vi "ACOPLADORES.vi"() -> ()   [LabVIEW 2014]
uses:
  <vilib>/Platform/TimedLoop/XDataNode/timing_clust.ctl
  <vilib>/Platform/TimedLoop/XDataNode/nitl_modes.ctl
  <vilib>/Platform/TimedLoop/XDataNode/wakeup.ctl
  <vilib>/Instr/_visa.llb/VISA Configure Serial Port (Instr).vi
  <vilib>/Platform/TimedLoop/XDataNode/XDataNode.xnode
  <userlib>/Newport ESP301/Newport ESP301.lvlib
  <vilib>/Platform/TimedLoop/XDataNode/XDNodeRunTimeDep.lvlib
panel:
  in  "Aceleração":dbl=300.0
  in  "D (um)":dbl=100.0
  in  "Raio":dbl=80.0
  in  "l int":dbl=50.0
  in  "Velocity":dbl=2.0
  out "PROGRESSÃO":i32=8
  in  "N_Guias":u32=8
  in  "Iniciar":bool
  in  "L":dbl=14.0 format="%.1f"
  in  "In.Curva":dbl=1.0
  in  "d (um)":dbl=7.0
  in  "Stop Button":bool
  out "X (mm)":dbl format="%.2g"
  out "Y (um)":dbl format="%.1f"
  out "XY Graph":cluster{dbl[], dbl[]}(graph)
  in  "Refresh Button":bool
  # "Tam.amostra (mm)"
  # "Núm.Acoplad."
  # "Inicio curva"
  # "Raio"
  # "D.Comp.Int. (um)"
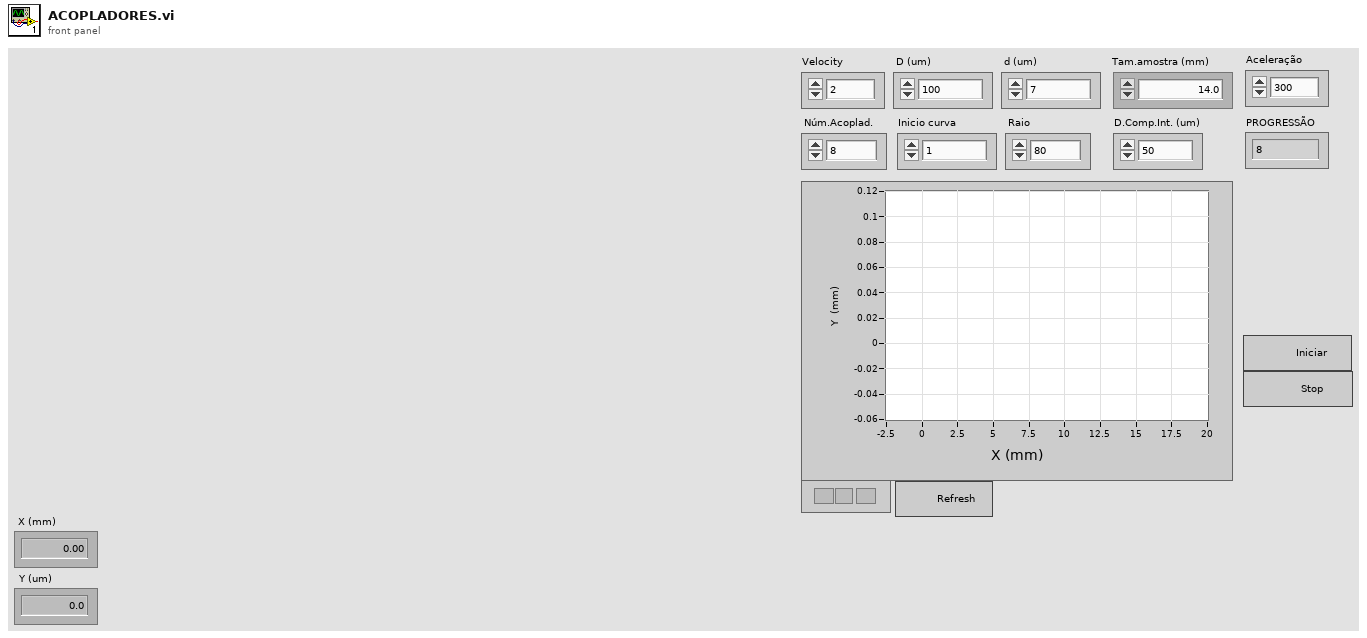
[diagram p1: front panel]
types:
  T1 = typedef "XDNodeRunTimeDep.lvlib/timing_clust.ctl" = cluster{"Expected End [f-1]":u64, "Actual End [f-1]":u64, "Finished Late? [f-1]":bool, "Expected End [i-1]":u64, "Actual End [i-1]":u64, "Finished Late? [i-1]":bool, "Expected Start [i]":u64, "Actual Start [i]":u64, "Expected Start [f]":u64, "Actual Start [f]":u64, "Source Name":string, "Structure Name":string, "Period":i64, "Deadline":i64, "Offset":i64, "Start":i64, "Priority":i32, "Timeout":i32, "Mode":T2, "Wakeup Reason":T3, "Error":errorcluster, "Source Type":string, "Secondary Source Type":string, "Global End Time":u64, "Global Start Time":u64, "Frame Duration":u64, "Iteration Duration":u64, "Assigned CPU":i32, "I/O Scan Engine Mode":u32}
  T2 = typedef "XDNodeRunTimeDep.lvlib/nitl_modes.ctl" = enum32{"No Change", "Process missed periods, maintain original phase", "Discard missed periods, maintain original phase", "Process missed periods, ignore original phase", "Discard missed periods, ignore original phase"}
  T3 = typedef "XDNodeRunTimeDep.lvlib/wakeup.ctl" = enum32{"Normal", "Aborted", "Asynchronous wakeup", "Timing source error", "Timed loop error", "Timeout"}
  T4 = cluster{"Axis1 moving":bool, "Axis2 moving":bool, "Axis3 moving":bool, "Axis4 moving":bool, "Motor Power of at least one axis":bool, "Reserved":bool, "Reserved":bool, "Reserved":bool, "Axis5 moving 2":bool, "Axis6 moving 2":bool, "Reserved":bool, "Reserved":bool, "Motor Power of at least one axis":bool, "Reserved":bool, "Reserved":bool, "Reserved":bool}
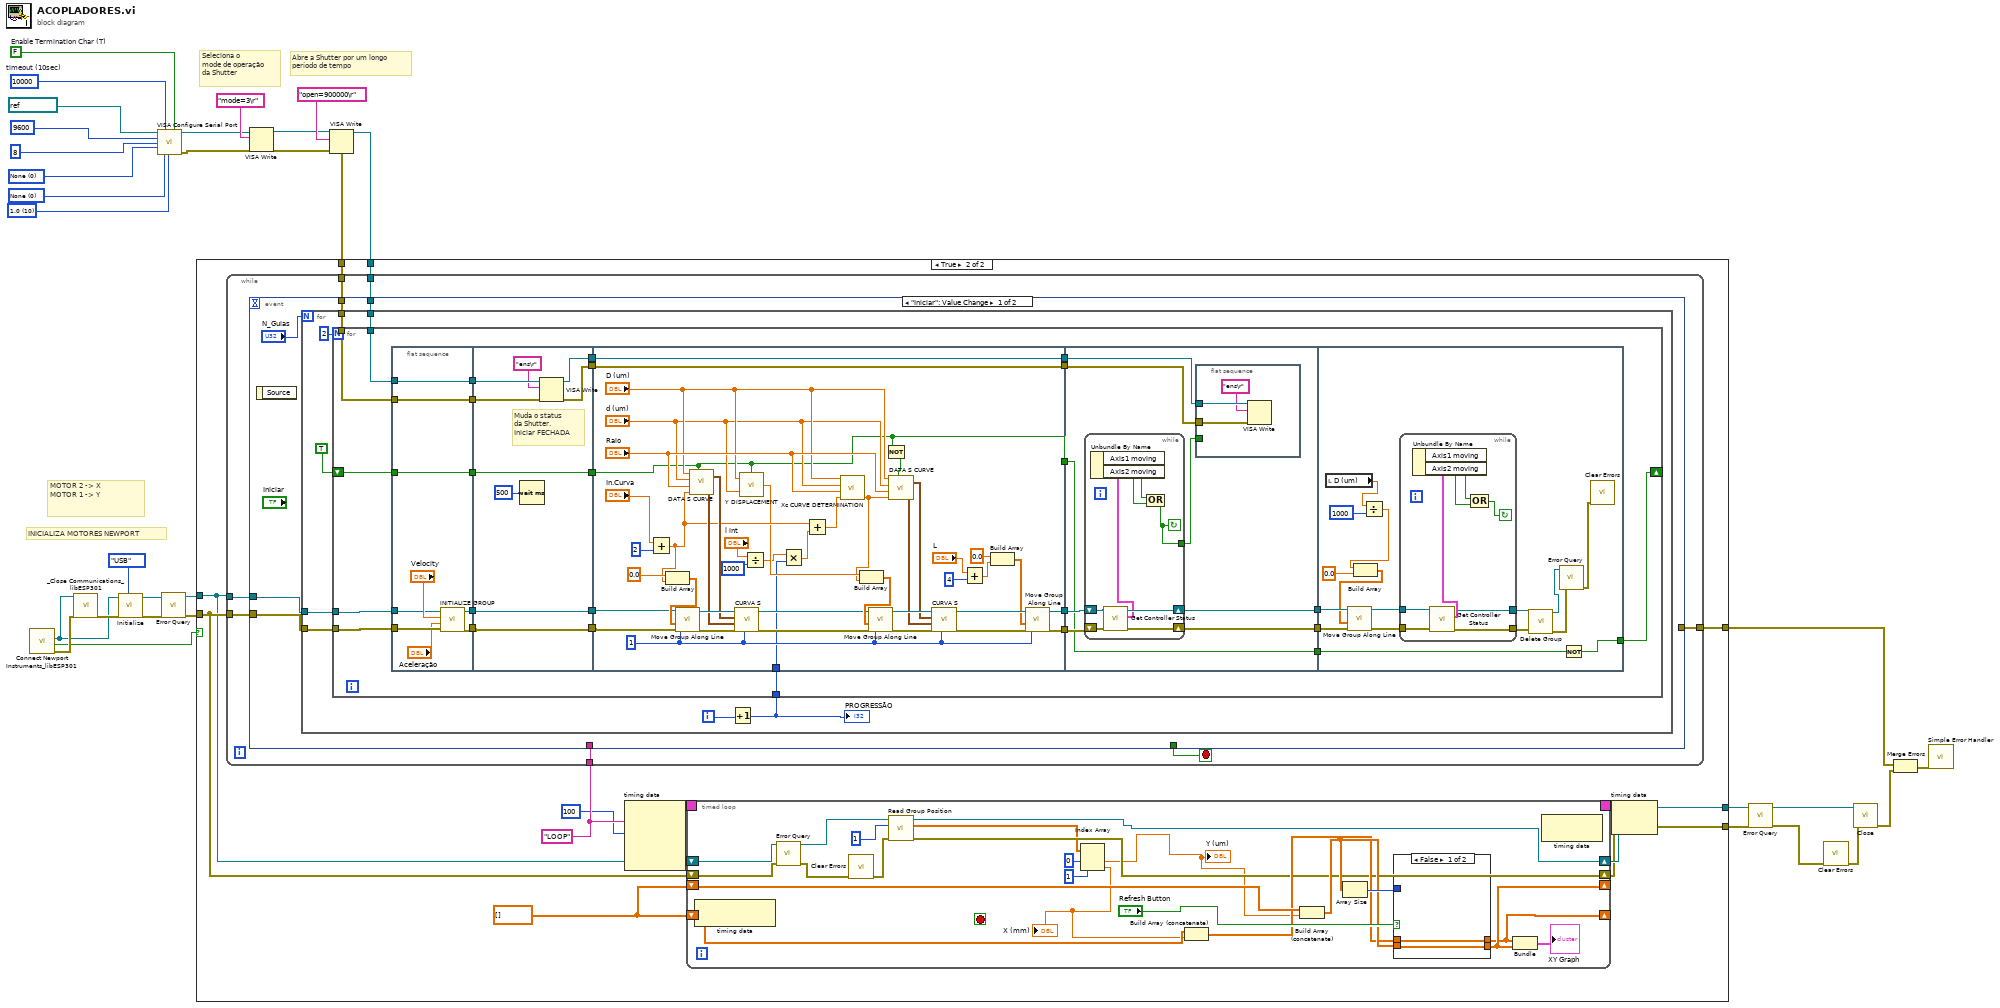
[diagram p0: block diagram]
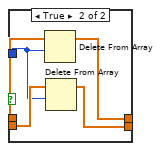
[diagram p3: hidden frame]
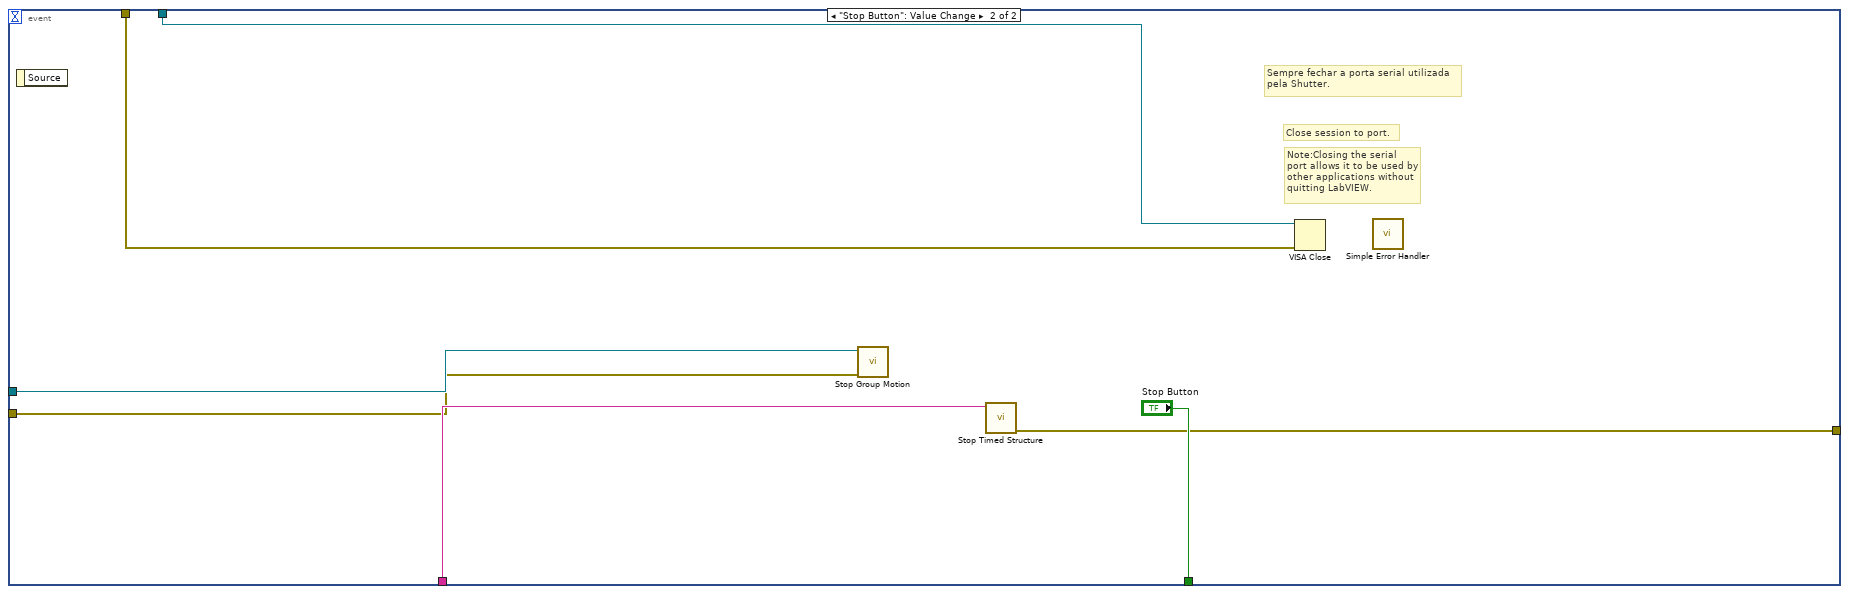
[diagram p4: hidden frame]
diagram:
  w9 = u16 0 items=["None", "Odd", "Even", "Mark", "Space"] ("parity")
  w12 = u16 10 items=["1.0"=10, "1.5"=15, "2.0"=20] ("stop bits")
  w13 = u16 0 items=["None"=0, "XON/XOFF"=1, "RTS/CTS"=2, "DTR/DSR"=4] ("flow control")
  w11 = FALSE  # Enable Termination Char (T)
  w10 = u32 10000  # timeout (10sec)
  # "Abre a Shutter por um longo\nperíodo de tempo"
  # "Seleciona o \nmode de operação\nda Shutter"
  # "MOTOR 2 -> X\nMOTOR 1 -> Y"
  # "INICIALIZA MOTORES NEWPORT"
  n1 = call <userlib>:"Connect Newport Instruments_libESP301.vi"() -> ("error (duplicate)"=w31:errorcluster, "Connected"=w20:bool, "VISA resource name (duplicate)"=w30:refnum<visa-resource-name>)  [unwired: 7 in, 2 out]
  n2 = call <userlib>:"_Close Communications_libESP301.vi"("Instrument Channel"=w30, "error in (no error)"=w31) -> ("error out"=w33:errorcluster)  [unwired: 13 in]
  n3 = call <userlib>:"Initialize.vi"("VISA resource name"=w30, "error in (no error)"=w33, "Serial Link (RS232)"=enum16{"RS232", "USB"}."USB") -> ("VISA resource name out"=w29:refnum<visa-resource-name>, "error out"=w28:errorcluster)  [unwired: 6 in]
  n4 = call-poly "VISA Configure Serial Port"("VISA resource name"=refnum<visa-resource-name> "COM6", "timeout (10sec)"=w10, "Enable Termination\nChar (T)"=w11, "baud rate (9600)"=u32 9600 ("baud rate"), "data bits (8)"=u16 8 ("data bits"), "parity (0:none)"=w9, "stop bits (10: 1 bit)"=w12, "flow control (0:none)"=w13) -> ("VISA resource name out"=w5:refnum<visa-resource-name>, "error out"=w4:errorcluster)  [unwired: 6 in]
  n5 = call <userlib>:"Error Query.vi"("error in (no error)"=w28, "VISA resource name"=w29) -> ("error out"=w17:errorcluster, "VISA resource name out"=w18:refnum<visa-resource-name>)  [unwired: 2 in, 2 out]
  n6 = VISA Write(VISA resource name=w5, write buffer="mode=3\r", error in (no error)=w4) -> (VISA resource name out=w2:refnum<visa-resource-name>, error out=w1:errorcluster)  [unwired: 1 out]
  n7 = VISA Write(VISA resource name=w2, write buffer="open=900000\r", error in (no error)=w1) -> (VISA resource name out=w21:refnum<visa-resource-name>, error out=w19:errorcluster)  [unwired: 1 out]
  n8 = case shown="True" w20 {
    tunnel: [w35 w47] -> w16
    tunnel: [w34 w46] -> w15
    tunnel: w18 -> [w35 w36]
    tunnel: w17 -> [w34 w37]
    tunnel: [_ w44] -> w24
    tunnel: w21 -> [_ w43]
    tunnel: w19 -> [_ w42]
    frame False {
    }
    frame True {
      w38 = dbl[] []
      w45 = "LOOP" ("Structure Name")
      n9 = while {
        tunnel: w37 -> [w90]
        tunnel: w36 -> [w89]
        tunnel: w45 -> [w87]
        tunnel: [w86] -> w44
        tunnel: w43 -> [w85]
        tunnel: w42 -> [w84]
        stop <- w88 stop-if-true
        n10 = event shown="[0] \"Iniciar\": Value Change" {
          selector: _ -> [_ _]
          dyn-events: _ -> [_ _]
          timeout: _ -> [_ _]
          tunnel: w90 -> [w95 w234]
          tunnel: w89 -> [w94 w235]
          tunnel: [_ "Stop Button"] -> w88
          tunnel: w87 -> [_ w238]
          tunnel: [_ w237] -> w86
          tunnel: w85 -> [w93 w236]
          tunnel: w84 -> [w92 w233]
          event "Iniciar": Value Change {
            n11 = event-data() -> ()  [unwired: 1 in, 1 out]
            n12 = for {
              N: "N_Guias" -> [_]
              tunnel: w95 -> [w103]
              tunnel: w94 -> [w102]
              tunnel: w93 -> [w101]
              tunnel: w92 -> [w100]
              i -> [w97]
              n13 = Increment(x=w97) -> (x+1=w96:i32)
              "PROGRESSÃO" <- w96
              n14 = for {
                N: 2 -> [_]
                tunnel: w103 -> [w126]
                tunnel: w102 -> [w125]
                tunnel: w101 -> [w124]
                tunnel: w100 -> [w117]
                shift-right: [w107] -> _
                shift-left: TRUE -> [w108]
                tunnel: w96 -> [w104]
                n15 = flat-sequence {
                  tunnel: w117 -> [w136]
                  tunnel: w124 -> [w137]
                  tunnel: w125 -> [w134]
                  tunnel: w126 -> [w133]
                  tunnel: [w132] -> w116
                  tunnel: [w131] -> w115
                  tunnel: [w137] -> w114
                  tunnel: [w136] -> w113
                  tunnel: [w130] -> w109
                  tunnel: w108 -> [w130]
                  tunnel: [w140] -> w128
                  tunnel: [w141] -> w127
                  tunnel: [w144] -> w121
                  tunnel: [w143] -> w119
                  tunnel: w116 -> [w140]
                  tunnel: w115 -> [w141]
                  tunnel: w114 -> [w145]
                  tunnel: w113 -> [w142]
                  tunnel: [w138] -> w110
                  tunnel: w109 -> [w138]
                  tunnel: w128 -> [w182]
                  tunnel: w127 -> [w183]
                  tunnel: w121 -> [w188]
                  tunnel: [w189] -> w120
                  tunnel: w119 -> [w189]
                  tunnel: [w188] -> w118
                  tunnel: [w155] -> w112
                  tunnel: [w154] -> w111
                  tunnel: w110 -> [w148]
                  tunnel: [w148] -> w105
                  tunnel: w104 -> [w153]
                  tunnel: [w197] -> w123
                  tunnel: [w196] -> w122
                  tunnel: w118 -> [w194]
                  tunnel: w120 -> [w195]
                  tunnel: w112 -> [w192]
                  tunnel: w111 -> [w191]
                  tunnel: [w190] -> w106
                  tunnel: w105 -> [w190]
                  tunnel: w123 -> [w217]
                  tunnel: w122 -> [w216]
                  tunnel: [w212] -> w107
                  tunnel: w106 -> [w213]
                  frame #0 {
                    n16 = call "INITIALIZE GROUP.vi"("error in (no error)"=w133, "Aceleração"="Aceleração", "Velocity"="Velocity", "VISA Refnum in"=w134) -> ("error out"=w132:errorcluster, "VISA Refnum out"=w131:refnum<visa-resource-name>)  [unwired: 6 in]
                  }
                  frame #1 {
                    # "Muda o status\nda Shutter.\nIniciar FECHADA"
                    n17 = Wait (ms)(milliseconds to wait=u32 500) -> ()  [unwired: 1 out]
                    n18 = VISA Write(VISA resource name=w145, write buffer="ens\r", error in (no error)=w142) -> (VISA resource name out=w144:refnum<visa-resource-name>, error out=w143:errorcluster)  [unwired: 1 out]
                  }
                  frame #2 {
                    w169 = 1
                    n19 = Add(x="In.Curva", y=u32 2) -> (x+y=w167:dbl)
                    n20 = Build Array(0.0 ("element"), w167) -> (w186:dbl[])
                    n21 = call <userlib>:"Move Group Along Line.vi"("error in (no error)"=w182, "Position (0 units)"=w186, "Group Number (1)"=w169, "VISA resource name"=w183) -> ("error out"=w180:errorcluster, "VISA resource name out"=w181:refnum<visa-resource-name>)  [unwired: 2 in]
                    n22 = call "DATA S CURVE.vi"("Distância Guias (um)"="D (um)", "Distância Ac (um)"="d (um)", "Raio"="Raio", "Xc"=w167, "Blank Button"=w148) -> ("1st curve"=w172:cluster{"Yc":dbl, "Xc":dbl, "Angle":dbl}, "2nd curve"=w171:cluster{"Yc":dbl, "Xc":dbl, "Angle":dbl})
                    n23 = call "CURVA S.vi"("VISA Refnum in"=w181, "1st curve parameters"=w172, "2nd curve parameters"=w171, "error in (no error)"=w180, "Grupo"=w169) -> ("VISA Refnum out"=w179:refnum<visa-resource-name>, "error out"=w178:errorcluster)
                    n24 = call "Y DISPLACEMENT.vi"("Desce ou sobe?"=w148, "Distância Ac (um)"="d (um)", "Distância Guias (um)"="D (um)") -> ("Delta Y"=w159:dbl)
                    n25 = Divide(x="l int", y=u32 1000) -> (x/y=w151:dbl)
                    n26 = Multiply(x=w151, y=w153) -> (x*y=w166:dbl)
                    n27 = Add(x=w167, y=w166) -> (x+y=w165:dbl)
                    n28 = call "Xc CURVE DETERMINATION.vi"("Deslocamento X"=w165, "Raio"="Raio", "Distância Ac (um)"="d (um)", "Distância Guias (um)"="D (um)") -> ("Xc"=w152:dbl)
                    n29 = Build Array(w159, w152) -> (w187:dbl[])
                    n30 = call <userlib>:"Move Group Along Line.vi"("error in (no error)"=w178, "Position (0 units)"=w187, "Group Number (1)"=w169, "VISA resource name"=w179) -> ("error out"=w176:errorcluster, "VISA resource name out"=w177:refnum<visa-resource-name>)  [unwired: 2 in]
                    n31 = Not(x=w148) -> (.not. x?=w147:bool)
                    n32 = call "DATA S CURVE.vi"("Distância Guias (um)"="D (um)", "Distância Ac (um)"="d (um)", "Raio"="Raio", "Xc"=w152, "Blank Button"=w147) -> ("1st curve"=w170:cluster{"Yc":dbl, "Xc":dbl, "Angle":dbl}, "2nd curve"=w164:cluster{"Yc":dbl, "Xc":dbl, "Angle":dbl})
                    n33 = call "CURVA S.vi"("VISA Refnum in"=w177, "1st curve parameters"=w170, "2nd curve parameters"=w164, "error in (no error)"=w176, "Grupo"=w169) -> ("VISA Refnum out"=w175:refnum<visa-resource-name>, "error out"=w174:errorcluster)
                    n34 = Add(x="L", y=u32 4) -> (x+y=w158:dbl)
                    n35 = Build Array(0.0 ("element"), w158) -> (w156:dbl[])
                    n36 = call <userlib>:"Move Group Along Line.vi"("error in (no error)"=w174, "Position (0 units)"=w156, "Group Number (1)"=w169, "VISA resource name"=w175) -> ("error out"=w154:errorcluster, "VISA resource name out"=w155:refnum<visa-resource-name>)  [unwired: 2 in]
                  }
                  frame #3 {
                    n37 = while {
                      shift-right: [w206] -> w196
                      shift-left: w192 -> [w208]
                      shift-right: [w205] -> w197
                      shift-left: w191 -> [w207]
                      tunnel: [w201] -> w193
                      stop <- w201 continue-if-true
                      n38 = call <userlib>:"Get Controller Status.vi"("error in (no error)"=w207, "VISA resource name"=w208) -> ("error out"=w205:errorcluster, "Controller Status"=w204:T4, "VISA resource name out"=w206:refnum<visa-resource-name>)  [unwired: 2 in, 1 out]
                      n39 = Unbundle By Name(w204) -> ("Axis1 moving"=w203:bool, "Axis2 moving"=w202:bool)
                      n40 = Compound Arithmetic op=OR(w203, w202) -> (w201:bool)
                    }
                    n41 = flat-sequence {
                      tunnel: w195 -> [w200]
                      tunnel: w194 -> [w199]
                      tunnel: w193 -> [_]
                      frame #0 {
                        n42 = VISA Write(VISA resource name=w199, write buffer="ens\r", error in (no error)=w200) -> ()  [unwired: 3 out]
                      }
                    }
                  }
                  frame #4 {
                    n43 = local read "D (um)"() -> (w210:dbl)
                    n44 = Divide(x=w210, y=u32 1000) -> (x/y=w209:dbl)
                    n45 = Build Array(w209, 0.0 ("element")) -> (w215:dbl[])
                    n46 = call <userlib>:"Move Group Along Line.vi"("error in (no error)"=w217, "Position (0 units)"=w215, "VISA resource name"=w216) -> ("error out"=w218:errorcluster, "VISA resource name out"=w219:refnum<visa-resource-name>)  [unwired: 3 in]
                    n47 = while {
                      tunnel: w219 -> [w228]
                      tunnel: w218 -> [w227]
                      tunnel: [w226] -> w224
                      tunnel: [w225] -> w223
                      stop <- w229 continue-if-true
                      n48 = call <userlib>:"Get Controller Status.vi"("error in (no error)"=w227, "VISA resource name"=w228) -> ("error out"=w225:errorcluster, "Controller Status"=w232:T4, "VISA resource name out"=w226:refnum<visa-resource-name>)  [unwired: 2 in, 1 out]
                      n49 = Unbundle By Name(w232) -> ("Axis1 moving"=w231:bool, "Axis2 moving"=w230:bool)
                      n50 = Compound Arithmetic op=OR(w231, w230) -> (w229:bool)
                    }
                    n51 = call <userlib>:"Delete Group.vi"("error in (no error)"=w223, "VISA resource name"=w224) -> ("error out"=w220:errorcluster, "VISA resource name out"=w221:refnum<visa-resource-name>)  [unwired: 4 in]
                    n52 = call <userlib>:"Error Query.vi"("error in (no error)"=w220, "VISA resource name"=w221) -> ("error out"=w222:errorcluster)  [unwired: 2 in, 3 out]
                    n53 = Not(x=w213) -> (.not. x?=w212:bool)
                    n54 = call <vilib>:"Clear Errors.vi"("error in (no error)"=w222) -> ()  [unwired: 5 in, 2 out]
                  }
                }
              }
            }
          }
          event "Stop Button": Value Change {
            # "Sempre fechar a porta serial utilizada\npela Shutter."
            # "Note:Closing the serial port allows it to be used by other applications without\nquitting LabVIEW."
            # "Close session to port."
            n55 = event-data() -> ()  [unwired: 1 in, 1 out]
            n56 = call <userlib>:"Stop Group Motion.vi"("error in (no error)"=w234, "VISA resource name"=w235) -> ()  [unwired: 4 in, 2 out]
            n57 = call <vilib>:"Stop Timed Structure.vi"("name"=w238) -> ("error out"=w237:errorcluster)  [unwired: 10 in]
            n58 = VISA Close(VISA resource name=w236, error in (no error)=w233) -> ()  [unwired: 1 out]
            n59 = call <vilib>:"Simple Error Handler.vi"() -> ()  [unwired: 5 in, 5 out]
          }
        }
      }
      n60 = node-c288(w45, i64 100 ("Period")) -> (w41:T1)  [unwired: 2 in]
      n61 = timed-loop {
        timing: w41 -> [_]
        timing-out: [_] -> w40
        shift-right: [w59] -> w47
        shift-left: w36 -> [w52]
        shift-right: [w58] -> w46
        shift-left: w37 -> [w51]
        shift-right: [w62] -> _
        shift-left: w38 -> [w66]
        shift-right: [w61] -> _
        shift-left: w38 -> [w64]
        stop <- _ stop-if-true
        n62 = node-c288() -> ()  [unwired: 1 in, 1 out]
        n63 = call <userlib>:"Error Query.vi"("error in (no error)"=w51, "VISA resource name"=w52) -> ("error out"=w49:errorcluster, "VISA resource name out"=w50:refnum<visa-resource-name>)  [unwired: 2 in, 2 out]
        n64 = call <vilib>:"Clear Errors.vi"("error in (no error)"=w49) -> ("error out"=w48:errorcluster)  [unwired: 5 in, 1 out]
        n65 = call <userlib>:"Read Group Position.vi"("error in (no error)"=w48, "Group Number (1)"=1, "VISA resource name"=w50) -> ("error out"=w58:errorcluster, "Position (units)"=w55:dbl[], "VISA resource name out"=w59:refnum<visa-resource-name>)  [unwired: 2 in]
        n66 = Index Array(array=w55, index #1=0 ("index"), index #2=1 ("index")) -> (element #1=w54:dbl, element #2=w53:dbl)
        "X (mm)" <- w53
        "Y (um)" <- w54
        n67 = Build Array (concatenate)(w64, w53) -> (w63:dbl[])
        n68 = Build Array (concatenate)(w66, w54) -> (w65:dbl[])
        n69 = Array Size(array=w65) -> (size(s)=w67:i32)
        n70 = case shown="False" "Refresh Button" {
          tunnel: [w71 w73] -> w61
          tunnel: w63 -> [w71 w76]
          tunnel: [w70 w72] -> w62
          tunnel: w65 -> [w70 w75]
          tunnel: w67 -> [_ w74]
          frame False {
          }
          frame True {
            n71 = Delete From Array(array=w76, length=w74) -> (array with subset deleted=w73:dbl[])  [unwired: 1 in, 1 out]
            n72 = Delete From Array(array=w75, length=w74) -> (array with subset deleted=w72:dbl[])  [unwired: 1 in, 1 out]
          }
        }
        n73 = Bundle(w61, w62) -> (→"XY Graph":cluster{dbl[], dbl[]})  [unwired: 1 in]
        n74 = node-c288() -> ()  [unwired: 1 in, 1 out]
      }
      n75 = node-c288(w40) -> ()  [unwired: 1 out]
    }
  }
  n76 = call <userlib>:"Error Query.vi"("error in (no error)"=w15, "VISA resource name"=w16) -> ("error out"=w25:errorcluster, "VISA resource name out"=w26:refnum<visa-resource-name>)  [unwired: 2 in, 2 out]
  n77 = call <vilib>:"Clear Errors.vi"("error in (no error)"=w25) -> ("error out"=w27:errorcluster)  [unwired: 5 in, 1 out]
  n78 = call <userlib>:"Close.vi"("error in (no error)"=w27, "VISA resource name"=w26) -> ("error out"=w23:errorcluster)  [unwired: 9 in]
  n79 = Merge Errors(w24, w23) -> (w22:errorcluster)
  n80 = call <vilib>:"Simple Error Handler.vi"("error in (no error)"=w22) -> ()  [unwired: 4 in, 5 out]
